vi "STM Write Meta Data (Serial Ref).vi"(6 "Options":T1={"Ignore Timeout Error"=TRUE, "timeout ms (1000)"=1000}, 7 "Meta data":T2[](array[typedef]), 8 "error in":errorcluster, 11 "VISA resource name":refnum<visa-resource-name>) -> (0 "error out":errorcluster, 3 "Connection Info Out":T3)   [LabVIEW 2013]
doc: "Use this VI to transmit the meta data cluster to a remote computer. Sending the meta data to another computer helps maintainability since the data resides only on one side and it is shared to other computers at run time."
uses:
  stm_Serial Connection Info.ctl
  stm_MetaDataElement.ctl
  stm_Serial Write Options.ctl
  Serial/Write Meta Data (Serial Clst).vi
  NI STM.lvlib
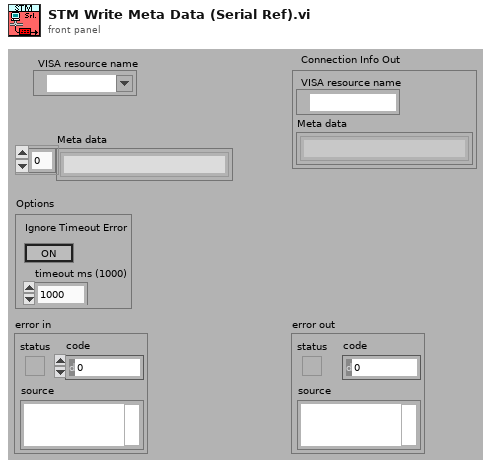
[diagram p1: front panel]
types:
  T1 = typedef "stm_Serial Write Options.ctl" = cluster{"Ignore Timeout Error":bool, "timeout ms (1000)":u32}
  T2 = typedef "stm_MetaDataElement.ctl" = string
  T3 = typedef "stm_Serial Connection Info.ctl" = cluster{"VISA resource name":refnum<visa-resource-name>, "Meta data":T2[]}
  T4 = typedef "NI STM.lvlib/Serial Connection Info.ctl" = cluster{"VISA resource name":refnum<visa-resource-name>, "meta data":T5[]}
  T5 = typedef "NI STM.lvlib/MetaDataElement.ctl" = string
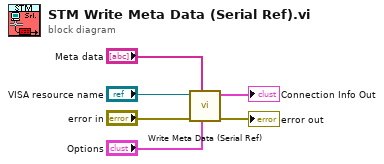
[diagram p0: block diagram]
diagram:
  n1 = call "Write Meta Data (Serial Ref).vi"("options"="Options", "meta data"="Meta data", "error in"="error in", "VISA resource name"="VISA resource name") -> ("error out"=→"error out":errorcluster, "connection info out"=→"Connection Info Out":T4)  [unwired: 6 in]
